vi "Thread_Display.vi"(8 "entrée d'erreur (pas d'erreur)":errorcluster, 11 "File d'attente en entrée":refnum<queue>) -> (0 "sortie d'erreur":errorcluster, 3 "File d'attente en sortie":refnum<queue>)   [LabVIEW 2020]
doc: "Thread Consommateur qui gère l'affichage"
uses:
  support/Message Queue/Message Cluster.ctl
  controls/UI Data.ctl
  support/Message Queue/All Message Queues.ctl
  Calculatrice/controls/ctrl_UI_Ref.ctl
  <vilib>/Utility/error.llb/Error Cluster From Error Code.vi
  <vilib>/ErrorRing/Error Ring.xnode
  support/Message Queue/Message Queue.lvlib
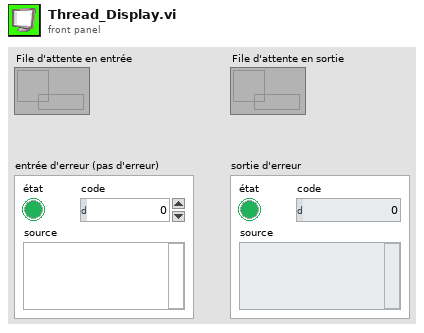
[diagram p1: front panel]
types:
  T1 = typedef "UI Data.ctl" = cluster{"Fifo":T2, "UI":T3, "Event":cluster{"Stop":refnum<user-event>}, "Data":cluster{"Display":cluster{"Num":dbl, "Char":string}, "memory":string}}
  T2 = typedef "Message Queue.lvlib/All Message Queues.ctl" = cluster{"Conductor":refnum<queue>, "IU":refnum<queue>}
  T3 = typedef "ctrl_UI_Ref.ctl" = cluster{"Display":refnum<vi>}
  T4 = cluster{"état":bool, "code":i32, "source":string}
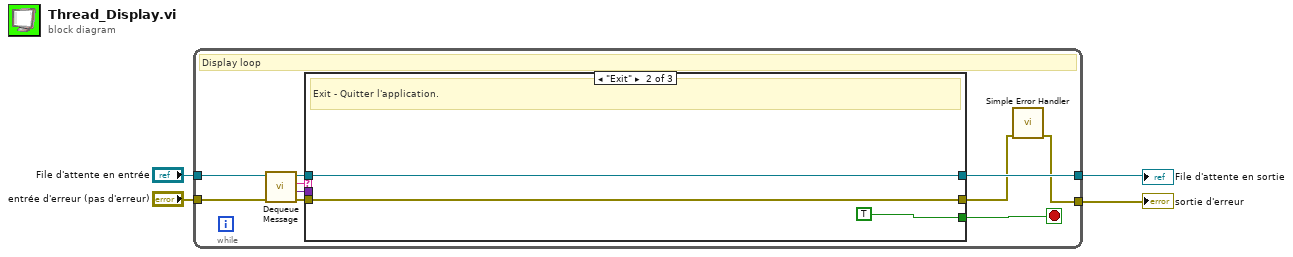
[diagram p0: block diagram]
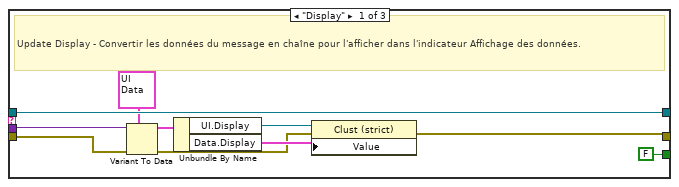
[diagram p2: hidden frame]
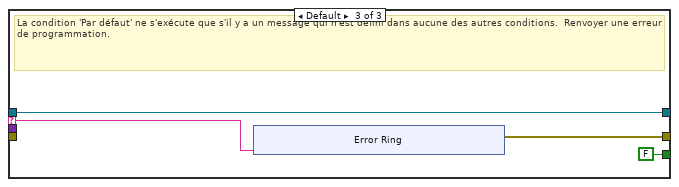
[diagram p3: hidden frame]
diagram:
  n1 = while {
    tunnel: "File d'attente en entrée" -> [w12]
    tunnel: "entrée d'erreur (pas d'erreur)" -> [w13]
    tunnel: [w5] -> w3
    tunnel: [w7] -> w4
    stop <- w14 stop-if-true
    # "Display loop"
    n2 = call "Dequeue Message.vi"("error in (no error)"=w13, "File d'attente de messages"=w12) -> ("error out"=w11:T4, "Données de message"=w9:variant, "Message"=w10:string, "File d'attente de message dup."=w8:refnum<queue>)  [unwired: 6 in]
    n3 = case "Conditions des messages" shown="\"Exit\"" w10 {
      selector: w10 -> [_ _ w30]
      tunnel: w8 -> [w23 w25 w28]
      tunnel: w11 -> [w22 w26 _]
      tunnel: [w15 w26 w31] -> w6
      tunnel: [FALSE TRUE FALSE] -> w14
      tunnel: w9 -> [w21 _ _]
      tunnel: [w23 w25 w28] -> w7
      frame "Display" {
        # "Update Display - Convertir les données du message en chaîne pour l'afficher dans l'indicateur Affichage des données."
        n4 = Variant To Data(error in=w22, type=T1 {"Fifo"={"Conductor"=refnum, "IU"=refnum}, "UI"={"Display"=refnum}, "Event"={"Stop"=refnum}, "Data"={"Display"={"Num"=0.0, "Char"=""}, "memory"=""}} ("Data Cluster"), Variant=w21) -> (data=w19:T1, error out=w16:errorcluster)
        n5 = Unbundle By Name(w19) -> ("UI.Display"=w18:refnum<vi>, "Data.Display"=w17:cluster{"Num":dbl, "Char":string})
        n6 = property class="Clust (strict)"(reference=w18, error in=w16, "Value"=w17) -> (error out=w15:errorcluster)  [unwired: 1 out]
      }
      frame "Exit" {
        # "Exit - Quitter l'application."
      }
      frame Default {
        # "La condition 'Par défaut' ne s'exécute que s'il y a un message qui n'est défini dans aucune des autres conditions.  Renvoyer une erreur de programmation."
        n7 = xnode ("Error Ring")("paramètre 0"=w30) -> ("sortie d'erreur"=w31:errorcluster)
      }
    }
    n8 = call <vilib>:"Simple Error Handler.vi"("error in (no error)"=w6) -> ("error out"=w5:errorcluster)  [unwired: 4 in, 4 out]
  }
  "File d'attente en sortie" <- w4
  "sortie d'erreur" <- w3
